vi "Is Vowel.vi"(1 "Single Character":string) -> (0 "Is Vowel?":bool)   [LabVIEW 2017]
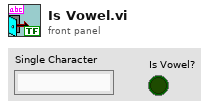
[diagram p1: front panel]
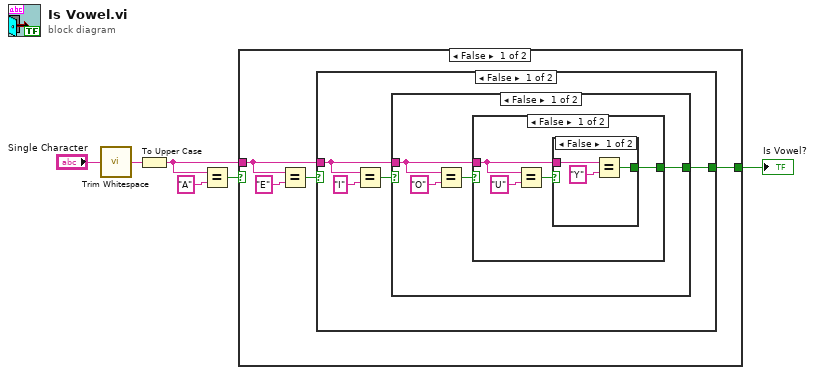
[diagram p0: block diagram]
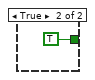
[diagram p2: hidden frame]
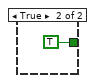
[diagram p3: hidden frame]
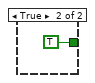
[diagram p4: hidden frame]
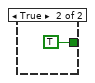
[diagram p5: hidden frame]
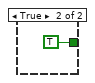
[diagram p6: hidden frame]
diagram:
  n1 = call <vilib>:"Trim Whitespace.vi"("string"="Single Character") -> ("trimmed string"=w1:string)  [unwired: 1 in]
  n2 = To Upper Case(1:w1) -> (0:w4:string)
  n3 = Equal?(x=w4, y="A") -> (x = y?=w5:bool)
  n4 = case shown="False" w5 {
    tunnel: w4 -> [w7 _]
    tunnel: [w8 TRUE ("Boolean")] -> w3
    frame False {
      n5 = Equal?(x=w7, y="E") -> (x = y?=w9:bool)
      n6 = case shown="False" w9 {
        tunnel: [w12 TRUE ("Boolean")] -> w8
        tunnel: w7 -> [w11 _]
        frame False {
          n7 = Equal?(x=w11, y="I") -> (x = y?=w13:bool)
          n8 = case shown="False" w13 {
            tunnel: [w16 TRUE ("Boolean")] -> w12
            tunnel: w11 -> [w15 _]
            frame False {
              n9 = Equal?(x=w15, y="O") -> (x = y?=w17:bool)
              n10 = case shown="False" w17 {
                tunnel: [w20 TRUE ("Boolean")] -> w16
                tunnel: w15 -> [w19 _]
                frame False {
                  n11 = Equal?(x=w19, y="U") -> (x = y?=w21:bool)
                  n12 = case shown="False" w21 {
                    tunnel: [w23 TRUE ("Boolean")] -> w20
                    tunnel: w19 -> [w24 _]
                    frame False {
                      n13 = Equal?(x=w24, y="Y") -> (x = y?=w23:bool)
                    }
                    frame True {
                    }
                  }
                }
                frame True {
                }
              }
            }
            frame True {
            }
          }
        }
        frame True {
        }
      }
    }
    frame True {
    }
  }
  "Is Vowel?" <- w3
